vi "Actor Core.vi"(8 "error in":errorcluster, 11 "ZWO_ASI in":refnum<class "ZWO_ASI.lvclass">) -> (0 "error out":errorcluster, 3 "Actor out":refnum<class "Actor.lvclass">)   [LabVIEW 2023, in "ZWO_ASI.lvlib" / "ZWO_ASI.lvclass"]
doc: "(<B>Filename</B>: Actor Framework.lvlib:Actor.lvclass:Actor Core.vi)\n\nReceives messages to the actor, reacts to them, and initiates any error handling that may shut the actor down.\n\nDescendant classes may override this VI to append parallel tasks for the actor to complete while it handles messages. Overrides use the Call Parent Class Method node."
uses:
  ZWO_ASI.lvclass
  ZWO_ASI.lvclass/ZWO_ASI.ctl
  <vilib>/ActorFramework/Actor/Actor.lvclass
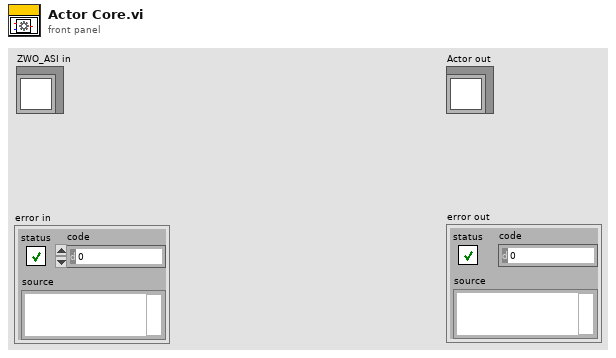
[diagram p1: front panel]
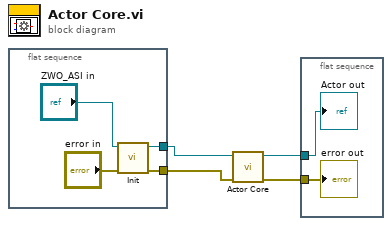
[diagram p0: block diagram]
diagram:
  n1 = flat-sequence {
    tunnel: [w7] -> w2
    tunnel: [w5] -> w1
    frame #0 {
      n2 = call-dynamic "Init.vi"("error in (no error)"="error in", "ZWO_ASI in"="ZWO_ASI in") -> ("error out"=w5:errorcluster, "ZWO_ASI out"=w7:refnum<class "ZWO_ASI.lvclass">)  [unwired: 8 in]
    }
  }
  n3 = call-parent "Actor Core.vi"("error in"=w1, "Actor in"=w2) -> ("error out"=w4:errorcluster, "Actor out"=w3:refnum<class "Actor.lvclass">)  [unwired: 8 in]
  n4 = flat-sequence {
    tunnel: w4 -> [w10]
    tunnel: w3 -> [w9]
    frame #0 {
      "error out" <- w10
      "Actor out" <- w9
    }
  }
